vi "FPGA_DAC_buses.vi"() -> ()   [LabVIEW 2010]
uses:
  <vilib>/rvi/DataTransferAndStorage/Container/XNode/niFpgaContainer.xnode
  <vilib>/rvi/FIFO/Fifo_Resource/nirvififoEmulationSetSize.vi
  <vilib>/rvi/DataTransferAndStorage/Container/Common/niFpgaContainerGetUniqueNameForEmu.vi
  <vilib>/rvi/Memory/Memory_Emulation/nirvimemoryEmulationManagerCache_GetValue.vi
  <vilib>/rvi/Memory/Memory_Emulation/nirvimemoryEmulationManagerCache_InsertValue.vi
  <vilib>/Utility/error.llb/Clear Errors.vi
  <vilib>/rvi/Memory/Memory_Emulation/nirvimemoryEmulationManagerCache_SetValue.vi
panel:
  in  "start movement":bool
  in  "buses to use":bool[](array[boolean])=[FALSE, FALSE, FALSE, FALSE, FALSE, FALSE, FALSE, FALSE]
  in  "wait(mSec)":u8
  in  "stop moving bus":bool
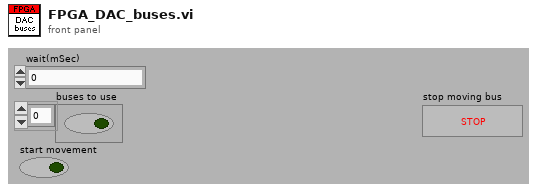
[diagram p1: front panel]
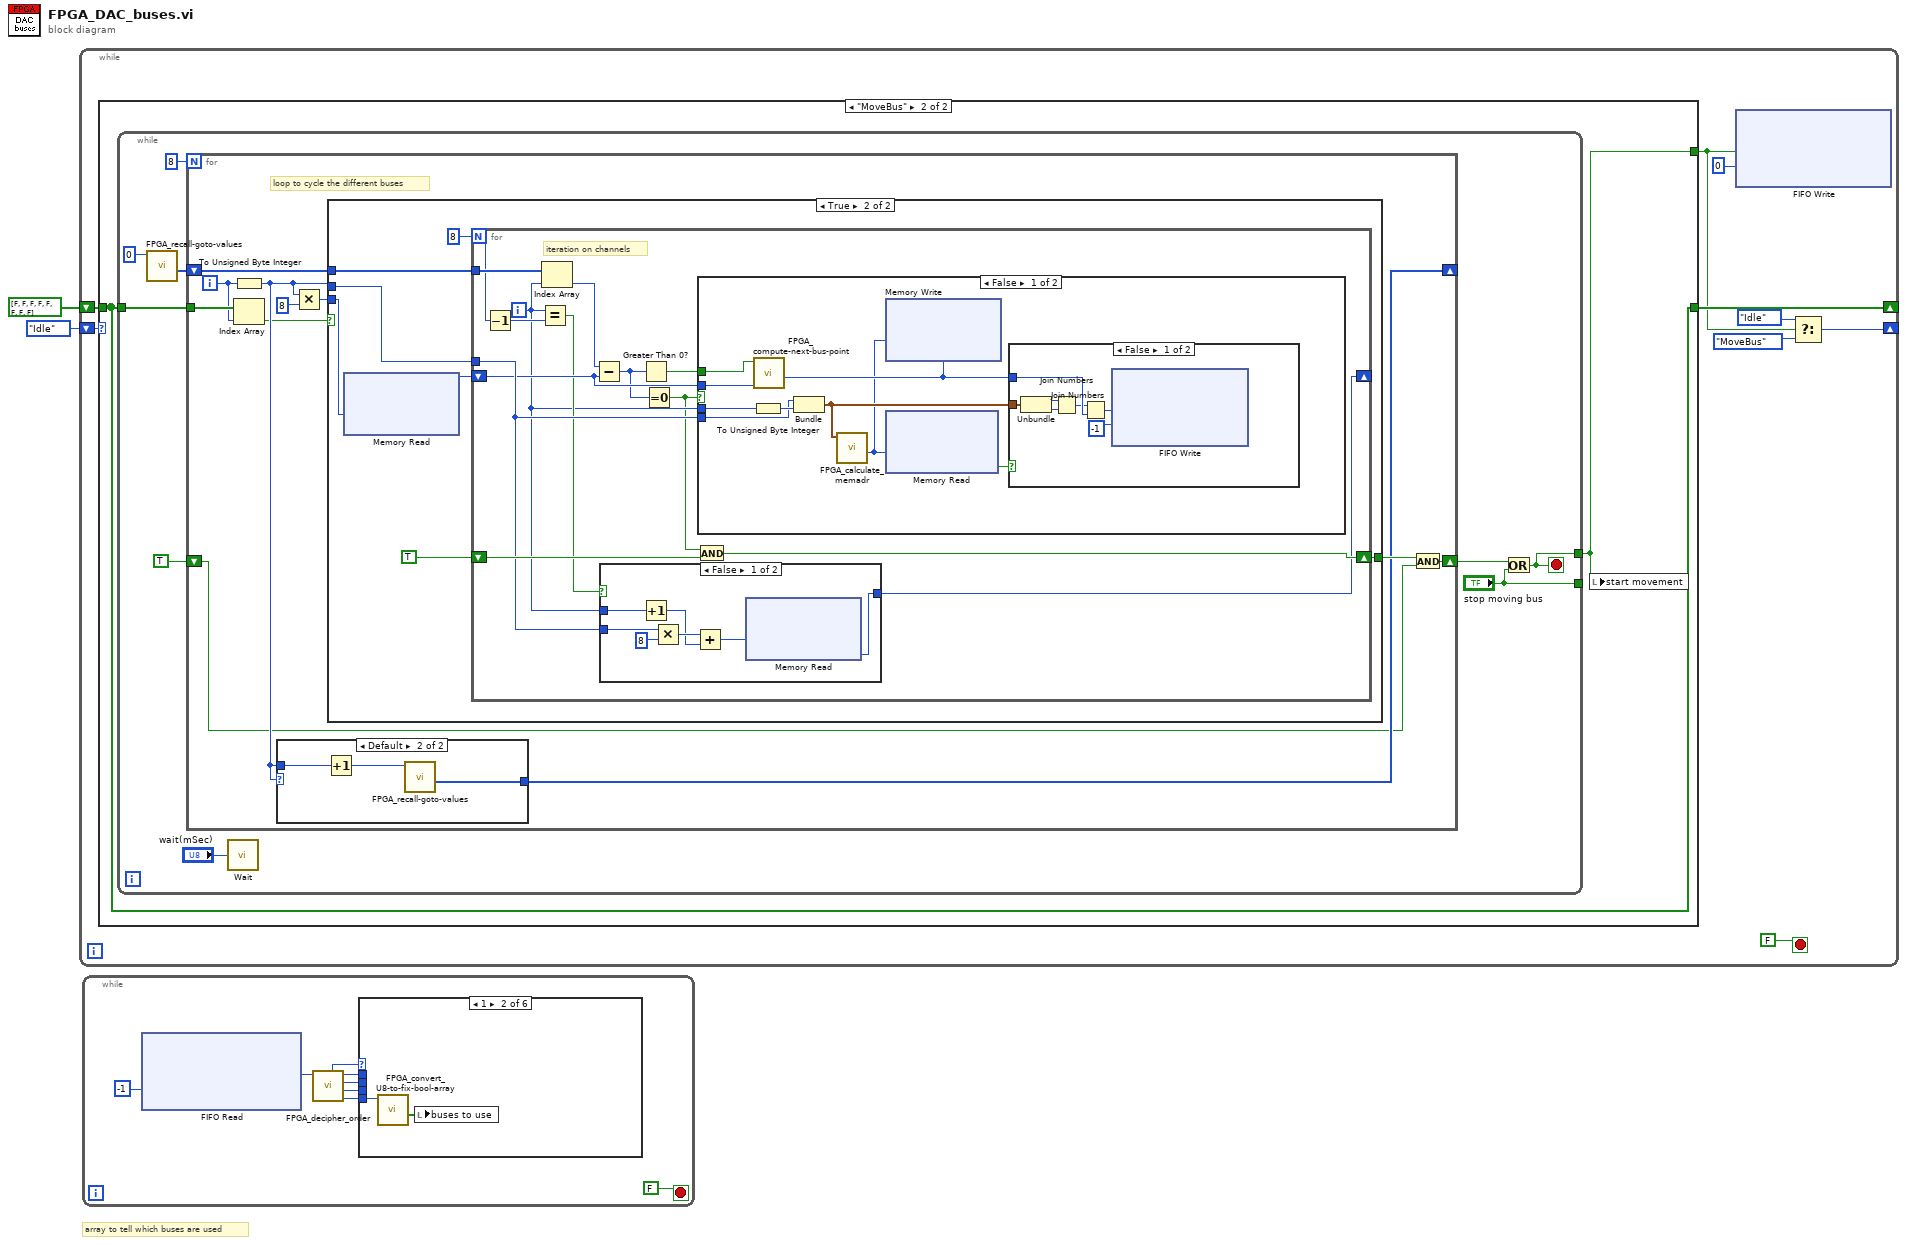
[diagram p0: block diagram]
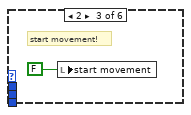
[diagram p3: hidden frame]
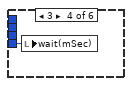
[diagram p4: hidden frame]
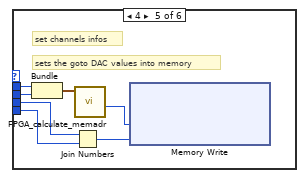
[diagram p5: hidden frame]
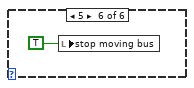
[diagram p6: hidden frame]
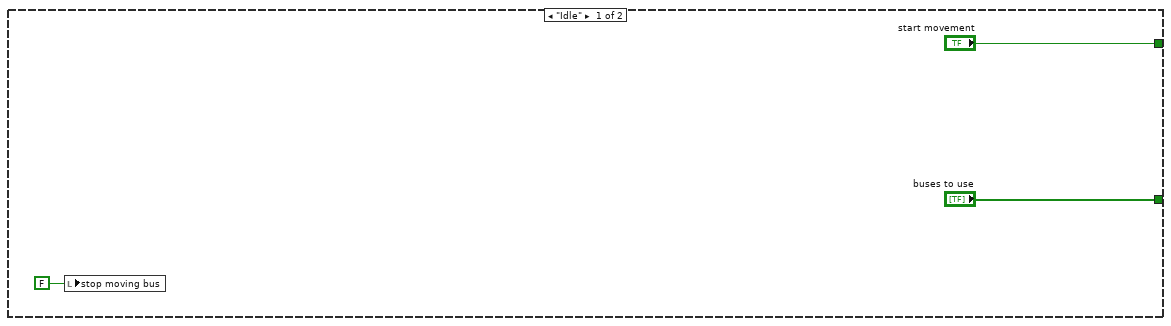
[diagram p7: hidden frame]
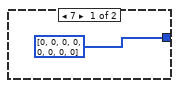
[diagram p8: hidden frame]
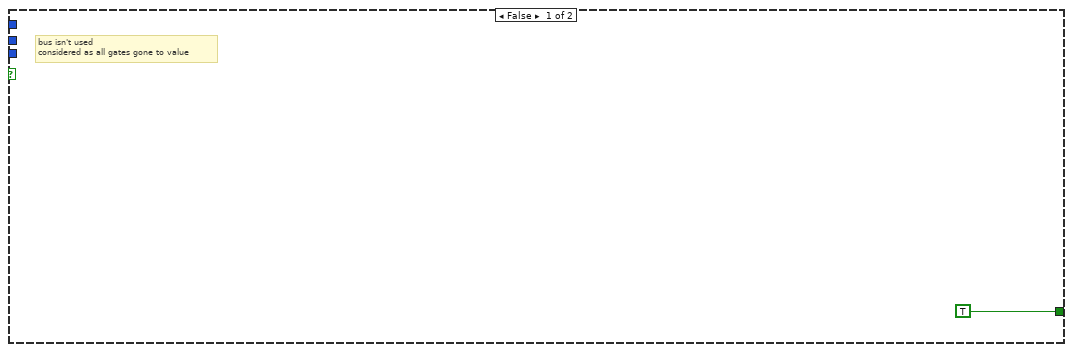
[diagram p9: hidden frame]
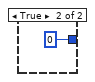
[diagram p10: hidden frame]
diagram:
  # "array to tell which buses are used"
  n1 = while {
    shift-right: [w8] -> _
    shift-left: enum16{"Idle", "MoveBus"}."Idle" -> [w11]
    shift-right: [w5] -> _
    shift-left: bool[] [FALSE, FALSE, FALSE, FALSE, FALSE, FALSE, FALSE, FALSE] -> [w6]
    stop <- FALSE stop-if-true
    n2 = case shown="\"MoveBus\"" w11 {
      tunnel: ["start movement" w66] -> w4
      tunnel: w6 -> [_ w67]
      tunnel: ["buses to use" w67] -> w5
      frame "Idle" {
        n3 = local write "stop moving bus"(FALSE ("stop moving bus")) -> ()
      }
      frame "MoveBus" {
        n4 = while {
          tunnel: ["stop moving bus"] -> _
          tunnel: [w75] -> w66
          tunnel: w67 -> [w71]
          stop <- w75 stop-if-true
          n5 = call "FPGA_recall-goto-values.vi"("panel"=u8 0) -> ("bus' goto values"=w69:u16[])  [unwired: 10 out]
          n6 = for {
            N: 8 -> [_]
            shift-right: [w86] -> w73
            shift-left: TRUE -> [w77]
            tunnel: w71 -> [w85]
            shift-right: [w81] -> _
            shift-left: w69 -> [w82]
            i -> [w78]
            # "loop to cycle the different buses"
            n7 = To Unsigned Byte Integer(number=w78) -> (unsigned 8bit integer=w80:u8)
            n8 = Index Array(array=w85, index=w78) -> (element=w79:bool)
            n9 = case shown="Default" w80 {
              tunnel: w80 -> [_ w91]
              tunnel: [u16[] [0, 0, 0, 0, 0, 0, 0, 0] ("bus' goto values") w89] -> w81
              frame 7 {
              }
              frame Default {
                n10 = Increment(x=w91) -> (x+1=w90:u8)
                n11 = call "FPGA_recall-goto-values.vi"("panel"=w90) -> ("bus' goto values"=w89:u16[])  [unwired: 10 out]
              }
            }
            n12 = Multiply(x=w80, y=u8 8) -> (x*y=w83:u8)
            n13 = case shown="True" w79 {
              tunnel: w82 -> [_ w96]
              tunnel: [TRUE w95] -> w87
              tunnel: w80 -> [_ w94]
              tunnel: w83 -> [_ w93]
              frame False {
                # "bus isn't used\nconsidered as all gates gone to value"
              }
              frame True {
                n14 = xnode ("Memory Read")("Address"=w93) -> ("Data"=w97:u16)  [unwired: 1 in, 1 out]
                n15 = for {
                  N: 8 -> [w233]
                  tunnel: w94 -> [w236]
                  tunnel: w96 -> [w239]
                  shift-right: [w237] -> w95
                  shift-left: TRUE -> [w238]
                  shift-right: [w234] -> _
                  shift-left: w97 -> [w235]
                  i -> [w229]
                  # "iteration on channels"
                  n16 = Decrement(x=w233) -> (x-1=w231:i32)
                  n17 = Equal?(x=w229, y=w231) -> (x = y?=w232:bool)
                  n18 = Index Array(array=w239, index=w229) -> (element=w230:u16)
                  n19 = Subtract(x=w230, y=w235) -> (x-y=w227:i32)
                  n20 = case shown="False" w232 {
                    tunnel: w236 -> [w246 _]
                    tunnel: w229 -> [w244 _]
                    tunnel: [w241 u16 0 ("Data")] -> w234
                    frame False {
                      n21 = Increment(x=w244) -> (x+1=w240:i32)
                      n22 = Multiply(x=w246, y=u8 8) -> (x*y=w245:u8)
                      n23 = Add(x=w245, y=w240) -> (x+y=w242:u8)
                      n24 = xnode ("Memory Read")("Address"=w242) -> ("Data"=w241:u16)  [unwired: 1 in, 1 out]
                    }
                    frame True {
                    }
                  }
                  n25 = Greater Than 0?(x=w227) -> (x > 0?=w226:bool)
                  n26 = Equal To 0?(x=w227) -> (x = 0?=w228:bool)
                  n27 = And(x=w228, y=w238) -> (x .and. y?=w237:bool)
                  n28 = case shown="False" w228 {
                    tunnel: w236 -> [w374 _]
                    tunnel: w229 -> [w375 _]
                    tunnel: w235 -> [w382 _]
                    tunnel: w226 -> [w378 _]
                    frame False {
                      n29 = To Unsigned Byte Integer(number=w375) -> (unsigned 8bit integer=w381:u8)
                      n30 = call "FPGA_compute-next-bus-point.vi"("channel actual"=w382, "increase value"=w378) -> ("next point"=w379:u16)  [unwired: 9 out]
                      n31 = Bundle(w374, w381) -> (w380:cluster{u8, u8})  [unwired: 1 out]
                      n32 = call "FPGA_calculate_memadr.vi"("Cluster"=w380) -> ("mem adr"=w376:u8)  [unwired: 10 out]
                      n33 = xnode ("Memory Write")("Address"=w376, "Data"=w379) -> ()  [unwired: 1 in, 1 out]
                      n34 = xnode ("Memory Read")("Address"=w376) -> ("Data"=w377:bool)  [unwired: 1 in, 1 out]
                      n35 = case shown="False" w377 {
                        tunnel: w380 -> [w639 _]
                        tunnel: w379 -> [w636 _]
                        frame False {
                          n36 = Unbundle(w639) -> (w637:u8, w638:u8)
                          n37 = Join Numbers(hi=w637, lo=w638) -> ((hi.lo)=w635:u16)
                          n38 = Join Numbers(hi=w635, lo=w636) -> ((hi.lo)=w634:u32)
                          n39 = xnode ("FIFO Write")("Element"=w634, "Timeout"=-1) -> ()  [unwired: 1 in, 2 out]
                        }
                        frame True {
                        }
                      }
                    }
                    frame True {
                    }
                  }
                }
              }
            }
            n40 = And(x=w87, y=w77) -> (x .and. y?=w86:bool)
          }
          n41 = call "Wait"("Count(mSec)"="wait(mSec)") -> ()  [unwired: 1 out]
          n42 = Or(x=w73, y="stop moving bus") -> (x .or. y?=w75:bool)
        }
        n43 = local write "start movement"(w66) -> ()
      }
    }
    n44 = xnode ("FIFO Write")("Element"=w4, "Timeout"=0) -> ()  [unwired: 1 in, 2 out]
    n45 = Select(t=enum16{"Idle", "MoveBus"}."Idle", s=w4, f=enum16{"Idle", "MoveBus"}."MoveBus") -> (s? t:f=w8:enum16{"Idle", "MoveBus"})
  }
  n46 = while {
    stop <- FALSE stop-if-true
    n47 = xnode ("FIFO Read")("Timeout"=-1) -> ("Element"=w699:u64)  [unwired: 1 in, 2 out]
    n48 = call "FPGA_decipher_order.vi"("order in"=w699) -> ("data 1"=w695:u8, "data 2"=w692:u8, "data 3"=w694:u8, "data 4"=w693:u8, "order out"=w696:u8)  [unwired: 6 out]
    n49 = case shown="1" w696 {
      tunnel: w695 -> [_ w752 _ w754 w756 _]
      tunnel: w694 -> [_ _ _ _ w759 _]
      tunnel: w693 -> [_ _ _ _ w758 _]
      tunnel: w692 -> [_ _ _ _ w755 _]
      frame 0, Default {
      }
      frame 1 {
        n50 = call "FPGA_convert_U8-to-fix-bool-array.vi"("U8"=w752) -> ("bool array"=w751:bool[])  [unwired: 10 out]
        n51 = local write "buses to use"(w751) -> ()
      }
      frame 2 {
        # "start movement!"
        n52 = local write "start movement"(FALSE ("start movement")) -> ()
      }
      frame 3 {
        n53 = local write "wait(mSec)"(w754) -> ()
      }
      frame 4 {
        # "sets the goto DAC values into memory"
        # "set channels infos"
        n54 = Bundle("data 4"=w758, "data 3"=w759) -> (w761:cluster{"data 4":u8, "data 3":u8})  [unwired: 1 out]
        n55 = Join Numbers(hi=w755, lo=w756) -> ((hi.lo)=w757:u16)
        n56 = call "FPGA_calculate_memadr.vi"("Cluster"=w761) -> ("mem adr"=w760:u8)  [unwired: 10 out]
        n57 = xnode ("Memory Write")("Address"=w760, "Data"=w757) -> ()  [unwired: 1 in, 1 out]
      }
      frame 5 {
        n58 = local write "stop moving bus"(TRUE ("stop moving bus")) -> ()
      }
    }
  }
